vi "AlliGator Get Ancillary Window Path.vi"(8 "Error In":errorcluster, 11 "AlliGator Window":T1=enum."Settings Window") -> (0 "Error Out":errorcluster, 3 "VI Path":path)   [LabVIEW 2021, in "AlliGator GUI.lvlib"]
doc: "Returns the path of the selected AlliGator window."
uses:
  AlliGator GUI.lvlib
  AlliGator Windows List.ctl
  AlliGator.vi
  Settings/AlliGator Settings Window.vi
  Dataset Information/Alligator Dataset Information Window.vi
  ROIs/AlliGator Source Image ROI Manager.vi
  ROIs/AlliGator Phasor Plot ROI Manager.vi
  Phasor Harmonic/AlliGator Phasor Harmonic Manager.vi
  Histograms/Histogram Window.vi
  Image Profile Window/AlliGator Source Image Profile Window.vi
  Local Decay Window/AlliGator Local Decay Window.vi
  About Alligator.vi
  Files/AlliGator Batch Dataset Export Window.vi
  Shot Noise Influence of Average Lifetime/AlliGator Shot Noise Influence on Average Lifetime.vi
  Fit Method Benchmark/AlliGator Fit Method Benchmark.vi
  Formula/Aliases Definition Window.vi
  Decay Fit Parameter Map/AlliGator Fit Results Constraints Window.vi
  Dataset Information/AlliGator Dataset Information Window.lvlib
  Notebook/Notebook.lvlib
  Settings/AlliGator Settings.lvlib
  ROIs/AlliGator ROIs.lvlib
  Phasor Harmonic/AlliGator Phasor Harmonics.lvlib
  Image Profile Window/AlliGator Image Profile Window.lvlib
  Files/AlliGator Files.lvlib
  Local Decay Window/AlliGator Local Decay Window.lvlib
  Histograms/Histogram Window.lvlib
  Shot Noise Influence of Average Lifetime/AlliGator Shot Noise Influence on Average Lifetime.lvlib
  Formula/Formula.lvlib
  Fit Method Benchmark/AlliGator Fit Method Benchmark.lvlib
  Decay Fit Parameter Map/AlliGator Decay Fit Parameter Map.lvlib
panel:
  # "see the AlliGator License on the block diagram (Ctrl+E or Window:Show Block Diagram)"
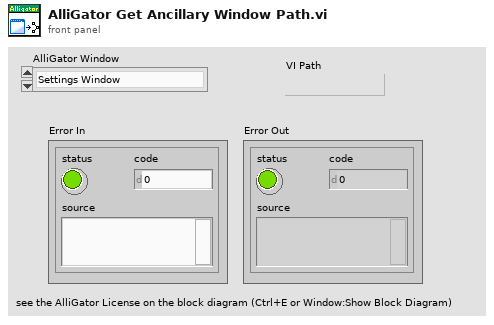
[diagram p1: front panel]
types:
  T1 = typedef "AlliGator GUI.lvlib/AlliGator Windows List.ctl" = enum16{"AlliGator Window", "Settings Window", "Notebook Window", "Dataset Information Window", "Source Image ROI Manager Window", "Phasor Plot ROI Manager Window", "Phasor Harmonic Manager Window", "Histogram Window", "Image Profile Window", "Local Decay Window", "About Window", "Batch Conversion Window", "Shot Noise Influence on Average Lifetime", "Fit Method Benchmark", "Camera Noise Influence on Lifetime", "AlliGator Alias Definition", "Fit Result Constraints Window"}
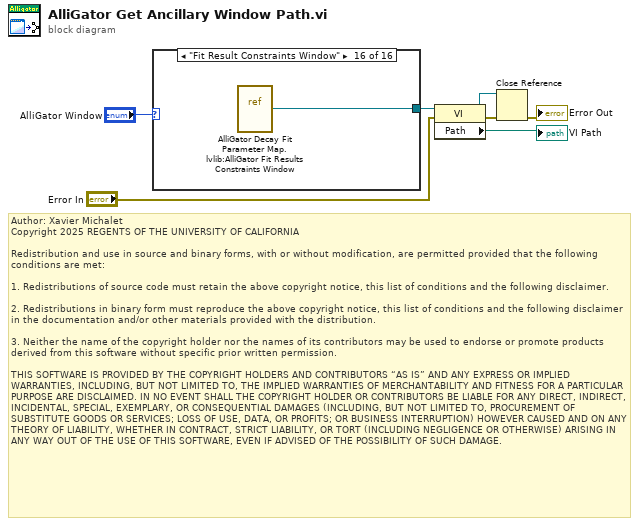
[diagram p0: block diagram]
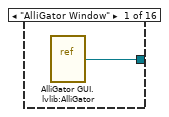
[diagram p2: hidden frame]
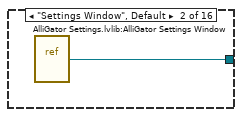
[diagram p3: hidden frame]
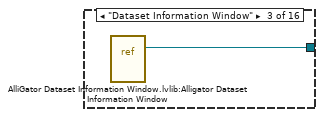
[diagram p4: hidden frame]
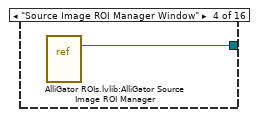
[diagram p5: hidden frame]
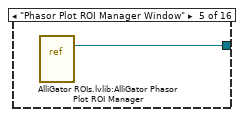
[diagram p6: hidden frame]
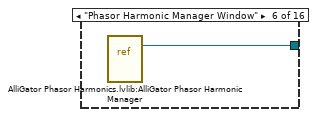
[diagram p7: hidden frame]
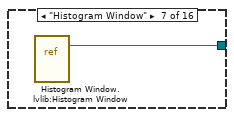
[diagram p8: hidden frame]
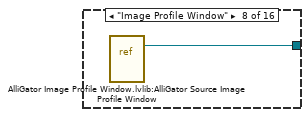
[diagram p9: hidden frame]
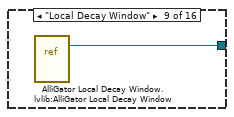
[diagram p10: hidden frame]
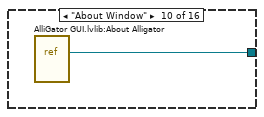
[diagram p11: hidden frame]
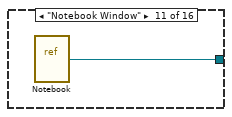
[diagram p12: hidden frame]
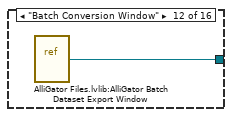
[diagram p13: hidden frame]
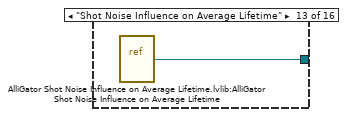
[diagram p14: hidden frame]
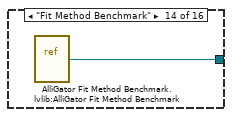
[diagram p15: hidden frame]
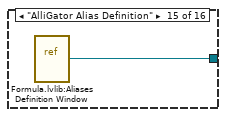
[diagram p16: hidden frame]
diagram:
  # "Author: Xavier Michalet\nCopyright 2025 REGENTS OF THE UNIVERSITY OF CALIFORNIA\n\nRedistribution and use in source and binary forms, with or without modification, are permitted provided that the following conditions are met:\n\n1. Redistributions of source code must retain the above copyright notice, this list of conditions and the following disclaimer.\n\n2. Redistributions in binary form must reproduce the above copyright notice, this list of conditions and the following disclaimer in the documentation and/or other materials provided with the distribution.\n\n3. Neither the name of the copyright holder nor the names of its contributors may be used to endorse or promote products derived from this software without specific prior written permission.\n\nTHIS SOFTWARE IS PROVIDED BY THE COPYRIGHT HOLDERS AND CONTRIBUTORS “AS IS” AND ANY EXPRESS OR IMPLIED WARRANTIES, INCLUDING, BUT NOT LIMITED TO, THE IMPLIED WARRANTIES OF MERCHANTABILITY AND FITNESS FOR A PARTICULAR PURPOSE ARE DISCLAIMED. IN NO EVENT SHALL THE COPYRIGHT HOLDER OR CONTRIBUTORS BE LIABLE FOR ANY DIRECT, INDIRECT, INCIDENTAL, SPECIAL, EXEMPLARY, OR CONSEQUENTIAL DAMAGES (INCLUDING, BUT NOT LIMITED TO, PROCUREMENT OF SUBSTITUTE GOODS OR SERVICES; LOSS OF USE, DATA, OR PROFITS; OR BUSINESS INTERRUPTION) HOWEVER CAUSED AND ON ANY THEORY OF LIABILITY, WHETHER IN CONTRACT, STRICT LIABILITY, OR TORT (INCLUDING NEGLIGENCE OR OTHERWISE) ARISING IN ANY WAY OUT OF THE USE OF THIS SOFTWARE, EVEN IF ADVISED OF THE POSSIBILITY OF SUCH DAMAGE."
  n1 = case shown="\"Fit Result Constraints Window\"" "AlliGator Window" {
    tunnel: [w8 w9 w10 w11 w12 w13 w14 w15 w16 w17 w18 w19 w20 w21 w22 w23] -> w6
    frame "AlliGator Window" {
      n2 = vi-ref "AlliGator GUI.lvlib:AlliGator.vi"() -> (w8:refnum<vi>)
    }
    frame "Settings Window", Default {
      n3 = vi-ref "AlliGator Settings.lvlib:AlliGator Settings Window.vi"() -> (w9:refnum<vi>)
    }
    frame "Dataset Information Window" {
      n4 = vi-ref "AlliGator Dataset Information Window.lvlib:Alligator Dataset Information Window.vi"() -> (w10:refnum<vi>)
    }
    frame "Source Image ROI Manager Window" {
      n5 = vi-ref "AlliGator ROIs.lvlib:AlliGator Source Image ROI Manager.vi"() -> (w11:refnum<vi>)
    }
    frame "Phasor Plot ROI Manager Window" {
      n6 = vi-ref "AlliGator ROIs.lvlib:AlliGator Phasor Plot ROI Manager.vi"() -> (w12:refnum<vi>)
    }
    frame "Phasor Harmonic Manager Window" {
      n7 = vi-ref "AlliGator Phasor Harmonics.lvlib:AlliGator Phasor Harmonic Manager.vi"() -> (w13:refnum<vi>)
    }
    frame "Histogram Window" {
      n8 = vi-ref "Histogram Window.lvlib:Histogram Window.vi"() -> (w14:refnum<vi>)
    }
    frame "Image Profile Window" {
      n9 = vi-ref "AlliGator Image Profile Window.lvlib:AlliGator Source Image Profile Window.vi"() -> (w15:refnum<vi>)
    }
    frame "Local Decay Window" {
      n10 = vi-ref "AlliGator Local Decay Window.lvlib:AlliGator Local Decay Window.vi"() -> (w16:refnum<vi>)
    }
    frame "About Window" {
      n11 = vi-ref "AlliGator GUI.lvlib:About Alligator.vi"() -> (w17:refnum<vi>)
    }
    frame "Notebook Window" {
      n12 = vi-ref "Notebook.vi"() -> (w18:refnum<vi>)
    }
    frame "Batch Conversion Window" {
      n13 = vi-ref "AlliGator Files.lvlib:AlliGator Batch Dataset Export Window.vi"() -> (w19:refnum<vi>)
    }
    frame "Shot Noise Influence on Average Lifetime" {
      n14 = vi-ref "AlliGator Shot Noise Influence on Average Lifetime.lvlib:AlliGator Shot Noise Influence on Average Lifetime.vi"() -> (w20:refnum<vi>)
    }
    frame "Fit Method Benchmark" {
      n15 = vi-ref "AlliGator Fit Method Benchmark.lvlib:AlliGator Fit Method Benchmark.vi"() -> (w21:refnum<vi>)
    }
    frame "AlliGator Alias Definition" {
      n16 = vi-ref "Formula.lvlib:Aliases Definition Window.vi"() -> (w22:refnum<vi>)
    }
    frame "Fit Result Constraints Window" {
      n17 = vi-ref "AlliGator Decay Fit Parameter Map.lvlib:AlliGator Fit Results Constraints Window.vi"() -> (w23:refnum<vi>)
    }
  }
  n18 = property class="VI"(reference=w6, error in="Error In") -> (reference out=w4:refnum<vi>, error out=w5:errorcluster, "Path"=→"VI Path":path)
  n19 = Close Reference(reference=w4, error in (no error)=w5) -> (error out=→"Error Out":errorcluster)
